vi "CLD 4 Event Structure Time Out Front Panel.vi"() -> ()   [LabVIEW 2019]
doc: "CLD 4 exercise"
panel:
  out "Time Has Elapsed":bool
  in  "Timeout Target (s)":dbl=2.0
  in  "Stop VI":bool
  in  "Decrement":bool
  out "Error Out":errorcluster
  in  "Error In":errorcluster
  out "Count":string="0"
  in  "Increment":bool
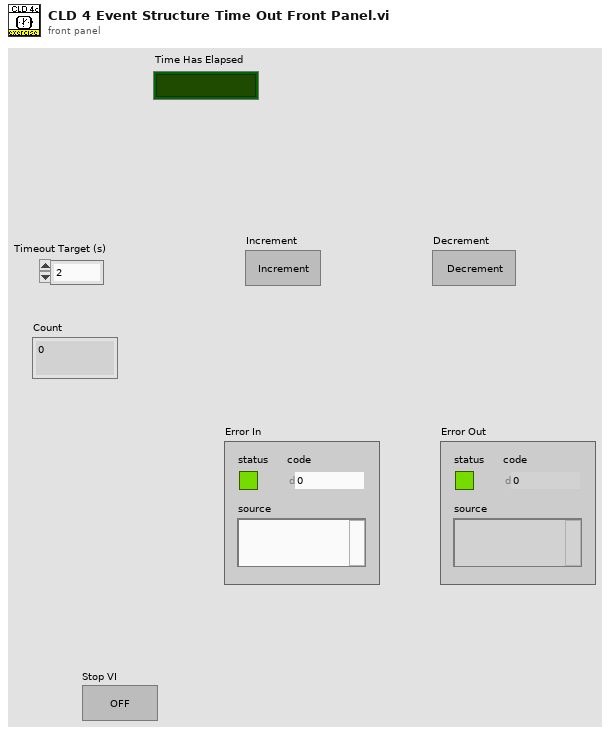
[diagram p1: front panel]
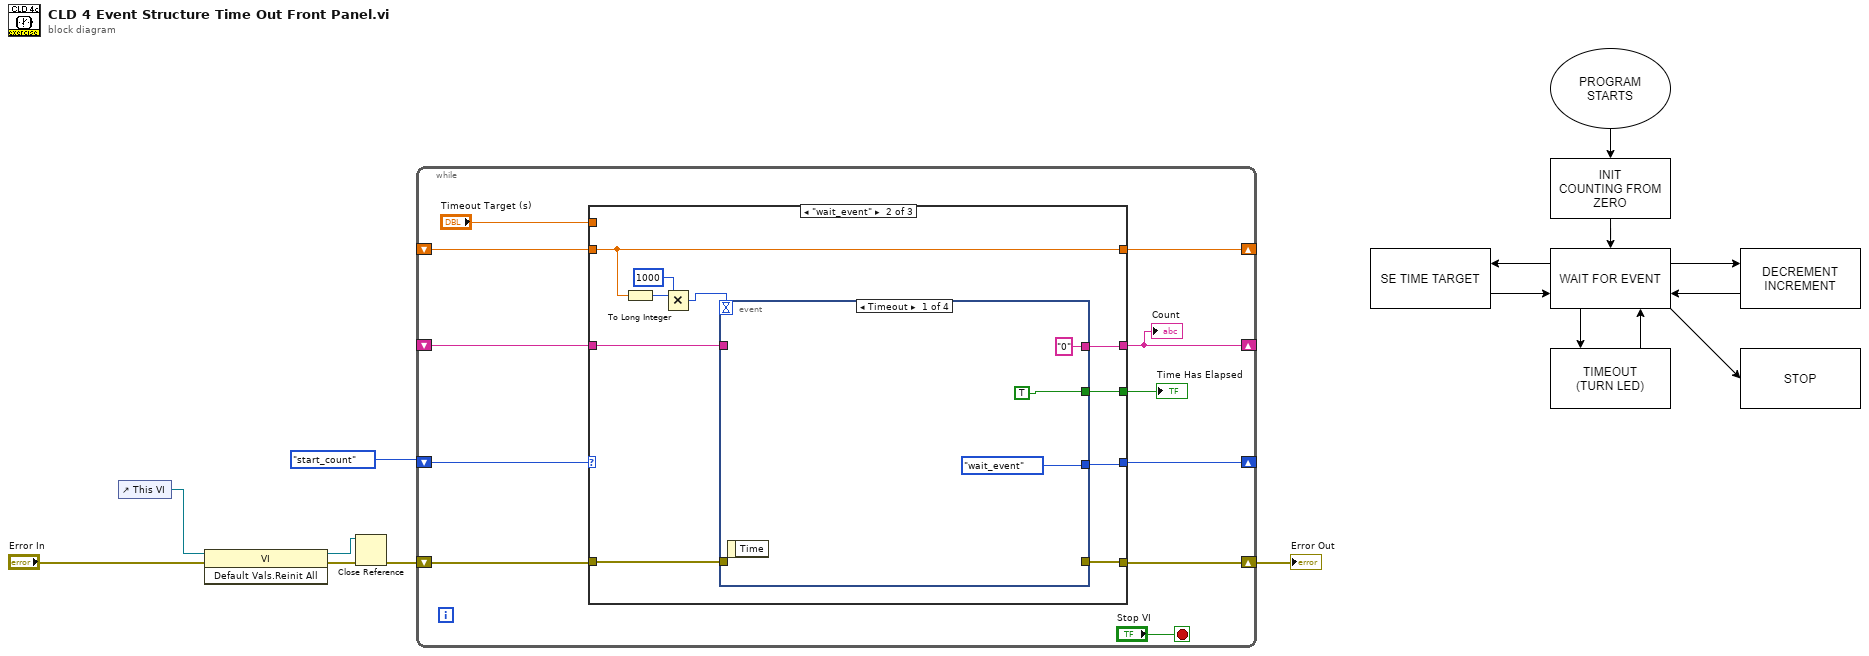
[diagram p0: block diagram]
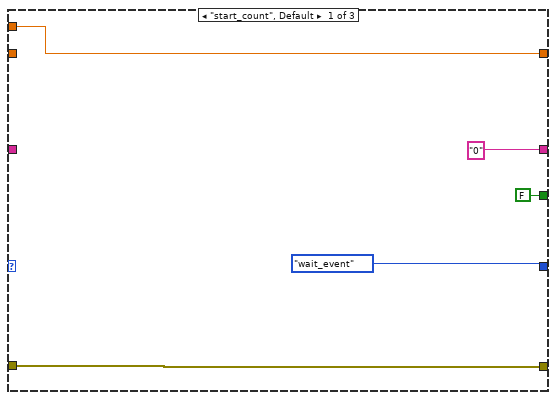
[diagram p2: hidden frame]
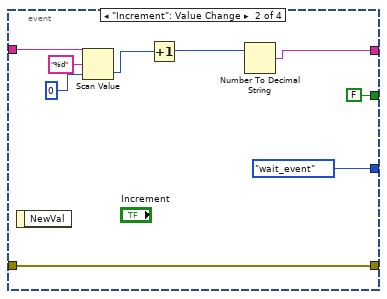
[diagram p3: hidden frame]
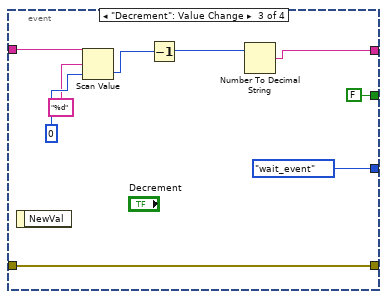
[diagram p4: hidden frame]
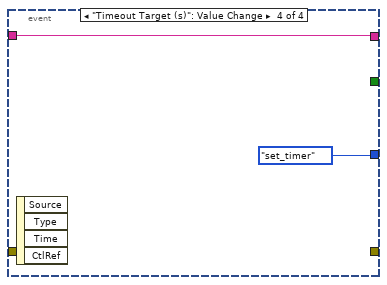
[diagram p5: hidden frame]
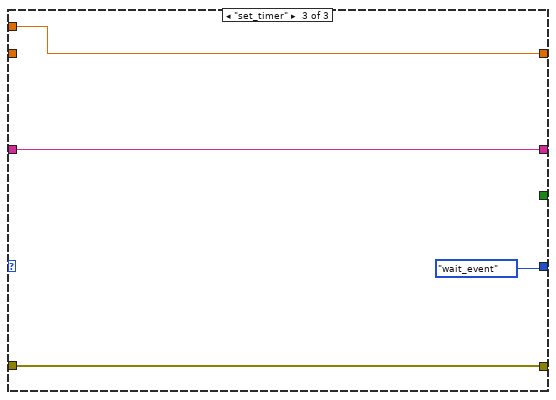
[diagram p6: hidden frame]
diagram:
  n1 = control-ref of="This VI"() -> (w4:refnum<vi>)
  n2 = invoke class="VI" method="Default Vals.Reinit All"(reference=w4, error in="Error In") -> (reference out=w3:refnum<vi>, error out=w5:errorcluster)  [unwired: 1 in, 1 out]
  n3 = Close Reference(reference=w3, error in (no error)=w5) -> (error out=w2:errorcluster)
  n4 = while {
    shift-right: [w17] -> w7
    shift-left: w2 -> [w12]
    shift-right: [w15] -> _
    shift-left: enum16{"start_count", "wait_event", "set_timer"}."start_count" -> [w16]
    shift-right: [w14] -> _
    shift-left: _ -> [w13]
    shift-right: [w10] -> _
    shift-left: _ -> [w9]
    stop <- "Stop VI" stop-if-true
    n5 = case shown="\"wait_event\"" w16 {
      tunnel: [w23 w32 w60] -> w17
      tunnel: w12 -> [w23 w33 w60]
      tunnel: [enum16{"start_count", "wait_event", "set_timer"}."wait_event" w29 enum16{"start_count", "wait_event", "set_timer"}."wait_event"] -> w15
      tunnel: ["0" ("Count") w30 w59] -> w14
      tunnel: w13 -> [_ w31 w59]
      tunnel: [FALSE ("Time Has Elapsed") w28 _] -> w11
      tunnel: w9 -> [_ w24 _]
      tunnel: [w19 w24 w58] -> w10
      tunnel: "Timeout Target (s)" -> [w19 _ w58]
      frame "start_count", Default {
      }
      frame "wait_event" {
        n6 = To Long Integer(number=w24) -> (32bit integer=w27:i32)
        n7 = Multiply(x=w27, y=1000) -> (x*y=w25:i32)
        n8 = event shown="[0] Timeout" {
          selector: _ -> [_ _ _ _]
          dyn-events: _ -> [_ _ _ _]
          timeout: w25 -> [_ _ _ _]
          tunnel: [_ w45 w54 _] -> w32
          tunnel: w33 -> [_ w45 w54 _]
          tunnel: w31 -> [_ w44 w53 w55]
          tunnel: ["0" ("Count") w40 w49 w55] -> w30
          tunnel: [enum16{"start_count", "wait_event", "set_timer"}."wait_event" enum16{"start_count", "wait_event", "set_timer"}."wait_event" enum16{"start_count", "wait_event", "set_timer"}."wait_event" enum16{"start_count", "wait_event", "set_timer"}."set_timer"] -> w29
          tunnel: [TRUE ("Time Has Elapsed") FALSE ("Time Has Elapsed") FALSE ("Time Has Elapsed") _] -> w28
          event Timeout {
            n9 = event-data() -> ()  [unwired: 1 in, 1 out]
          }
          event "Increment": Value Change {
            n10 = event-data() -> ()  [unwired: 1 in, 1 out]
            n11 = Scan Value(string=w44, format string="%d", default (0 dbl)=0 ("number")) -> (value=w43:i32)  [unwired: 1 out]
            n12 = Increment(x=w43) -> (x+1=w41:i32)
            n13 = Number To Decimal String(number=w41) -> (decimal integer string=w40:string)  [unwired: 1 in]
          }
          event "Decrement": Value Change {
            n14 = event-data() -> ()  [unwired: 1 in, 1 out]
            n15 = Scan Value(string=w53, format string="%d", default (0 dbl)=0 ("number")) -> (value=w52:i32)  [unwired: 1 out]
            n16 = Decrement(x=w52) -> (x-1=w50:i32)
            n17 = Number To Decimal String(number=w50) -> (decimal integer string=w49:string)  [unwired: 1 in]
          }
          event "Timeout Target (s)": Value Change {
            n18 = event-data() -> ()  [unwired: 1 in, 4 out]
          }
        }
      }
      frame "set_timer" {
      }
    }
    "Count" <- w14
    "Time Has Elapsed" <- w11
  }
  "Error Out" <- w7
